vi "C-IV.vi"(5 "save?":bool=TRUE, 7 "Remote Lockin Address":string, 8 "error in":errorcluster, 9 "Experiment Comments":string="SA03036H\nsweep Vsg:-150mV to 600mV, 1mV steps\nB: 7T to -7T\nVbg = -3.9V\nT: 50mK\n\nlockin\n\nI+/-: 2/3 3mV ac+ 250uV dc bias, 0.4 Hz\nV1+/-: 8/4\nV2+/- 6/28\nV3+/V3-: 27/8\nVsg: 1\nVbg :26\n\ntc 300ms order 2", 10 "Experiment folder name":string="6H_IVcurves", 11 "SweepControl.lvclass":refnum<class "SweepControl.lvclass">) -> (0 "error out":errorcluster, 3 "SweepControl out":refnum<class "SweepControl.lvclass">)   [LabVIEW 2016, in "Transport.lvclass"]
uses:
  Transport.lvclass
  SweepControl/SweepControl.lvclass
  <userlib>/LevyLab/Lockin-Multichannel/Instrument.Lockin/Typedefs/AO-cluster.ctl
  <userlib>/LevyLab/Lockin-Multichannel/Instrument.Lockin/Typedefs/AO_Amp-array.ctl
  <userlib>/LevyLab/Lockin-Multichannel/Instrument.Lockin/Typedefs/AO_DC-array.ctl
  <userlib>/LevyLab/Lockin-Multichannel/Instrument.Lockin/Typedefs/AO_f-array.ctl
  <userlib>/LevyLab/Lockin-Multichannel/Instrument.Lockin/Typedefs/AO_phi-array.ctl
  <userlib>/LevyLab/Lockin-Multichannel/Instrument.Lockin/Typedefs/Function-array.ctl
  <userlib>/LevyLab/Lockin-Multichannel/Instrument.Lockin/Typedefs/Function-enum.ctl
  <userlib>/LevyLab/LV to ITX/LVtoITX.lvclass
  Control Experiment/Control Experiment.lvclass
  <userlib>/LevyLab/Lockin-Multichannel/Instrument.Lockin/Instrument.Lockin.lvclass
panel:
  out "4Term":cluster{dbl[], dbl[]}[](graph)
  out "2Term":T1(graph)
  in  "Tab Control":T2(tab)
  in  "Channels: AO":T3={"AO Amp (V)"=[0.01, 0.0, 0.0, 0.0, 0.0, 0.0, 0.0, 0.0], "AO DC (V)"=[0.0, 0.0, 0.0, 0.0, 0.0, 0.0, 0.0, 0.0], "AO f (Hz)"=[13.1, 13.0, 13.0, 13.0, 13.0, 13.0, 13.0, 13.0], "AO Phase (°)"=[0.0, 0.0, 0.0, 0.0, 0.0, 0.0, 0.0, 0.0], "Function"=[enum."Sine", enum."Sine", enum."Sine", enum."Sine", enum."Sine", enum."Sine", enum."Sine", enum."Sine"], "I+"=[], "Sweeping"=[]} {"AO f (Hz)" min=0.001 max=10000.0; "AO DC (V)" format="%.3p"; "AO Amp (V)" format="%.3p"}
  in  "Source Channel":i32
  in  "decimating factor":i32=1
  in  "low cutoff freq: fl":dbl=0.01 format="%0.4f"
  out "Temp":dbl
  in  "offset":dbl[](array[numeric])=[0.0, 0.0, 0.0, 0.0, 0.0, 0.0] format="%_6p"
  in  "invert":dbl[](array[numeric])=[1.0, 1.0, 1.0, 1.0, 1.0, 1.0] format="%#_6p"
  out "DC Voltages":dbl[](array[numeric])=[0.00025, 0.3, 0.0, 0.0, 0.0, 0.0, 0.0, 0.0, 0.00025, 0.3, 0.0, 0.0, 0.0, 0.0, 0.0, 0.0, 0.00025, 0.3, 0.0, 0.0, 0.0, 0.0, 0.0, 0.0, 0.00025, 0.3, 0.0, 0.0, 0.0, 0.0, 0.0, 0.0, 0.00025, 0.3, 0.0, 0.0, 0.0, 0.0, 0.0, 0.0, 0.00025, 0.3, 0.0, 0.0, 0.0, 0.0, 0.0, 0.0, 0.00025, 0.3, 0.0, 0.0, 0.0, 0.0, 0.0, 0.0, 0.00025, 0.3, 0.0, 0.0, 0.0, 0.0, 0.0, 0.0]
  out "Field (T)":dbl
  in  "Current":i32=1 min=1
  in  "V1":i32=1 min=1
  in  "V2":i32=1 min=1
  out "Input signal":waveform(dbl)[](graph)
  out "output":dbl[][](graph)
  # "CONFIGURE TO READ B FIELD AND TEMPERATURE!!!!"
  # "1"
  # "2"
  # "3"
  # "4"
  # "5"
  # "6"
  # "7"
  # "8"
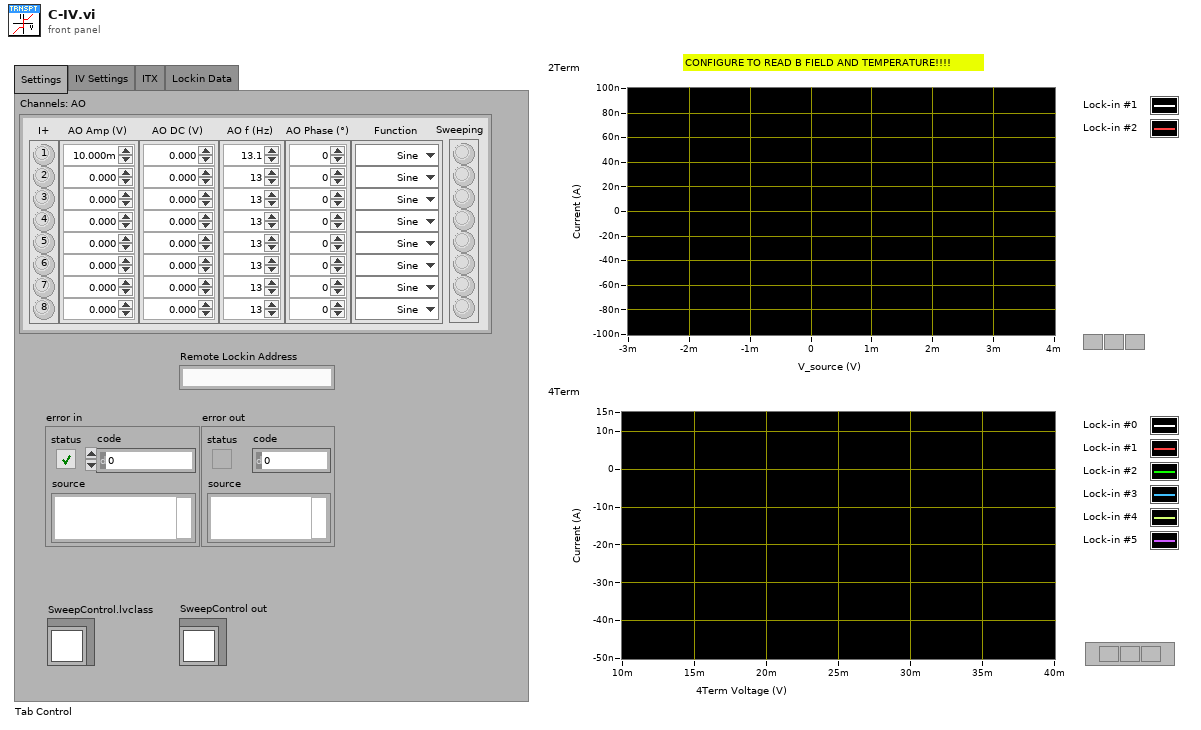
[diagram p1: front panel]
types:
  T1 = cluster{"Decimated and Filtered Array":dbl[], "Decimated and Filtered Array":dbl[]}[]
  T2 = enum32{"Settings", "IV Settings", "ITX", "Lockin Data"}
  T3 = typedef "Instrument.Lockin.lvclass/AO-cluster.ctl" = cluster{"AO Amp (V)":T4, "AO DC (V)":T5, "AO f (Hz)":T6, "AO Phase (°)":T7, "Function":T8, "I+":bool[], "Sweeping":bool[]}
  T4 = typedef "Instrument.Lockin.lvclass/AO_Amp-array.ctl" = dbl[]
  T5 = typedef "Instrument.Lockin.lvclass/AO_DC-array.ctl" = dbl[]
  T6 = typedef "Instrument.Lockin.lvclass/AO_f-array.ctl" = dbl[]
  T7 = typedef "Instrument.Lockin.lvclass/AO_phi-array.ctl" = dbl[]
  T8 = typedef "Instrument.Lockin.lvclass/Function-array.ctl" = T9[]
  T9 = typedef "Instrument.Lockin.lvclass/Function-enum.ctl" = enum16{"Sine", "Triangle", "Square", "Sawtooth"}
  T10 = cluster{"Decimated and Filtered Array":dbl[], "Decimated and Filtered Array":dbl[]}
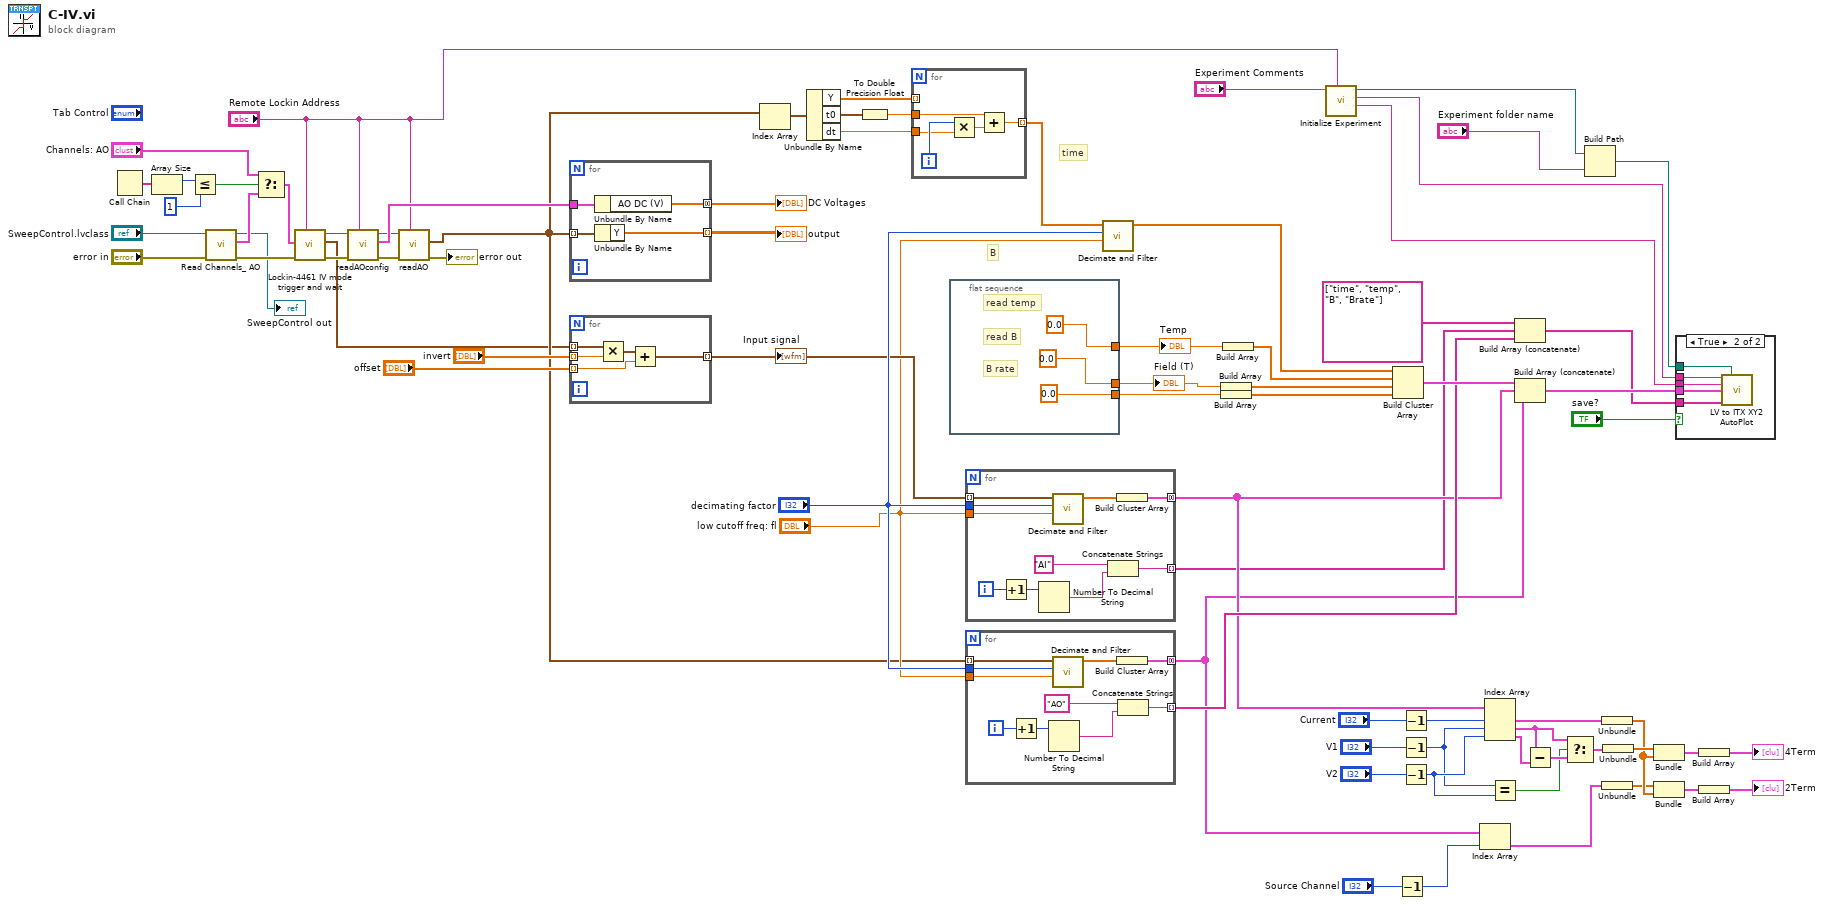
[diagram p0: block diagram]
diagram:
  # "time"
  # "B"
  n1 = Call Chain() -> (call chain=w35:string[])
  n2 = Array Size(array=w35) -> (size(s)=w34:i32)
  n3 = Less Or Equal?(x=w34, y=1) -> (x <= y?=w31:bool)
  n4 = call-dynamic "Read Channels_ AO.vi"("error in (no error)"="error in", "SweepControl in"="SweepControl.lvclass") -> ("error out"=w62:errorcluster, "Channels: AO"=w30:T3, "SweepControl out"=→"SweepControl out":refnum<class "SweepControl.lvclass">)  [unwired: 7 in]
  n5 = Select(t="Channels: AO", s=w31, f=w30) -> (s? t:f=w1:T3)
  n6 = call <userlib>:"Lockin-4461 IV mode trigger and wait.vi"("address"="Remote Lockin Address", "error in (no error)"=w62, "Channels: AO"=w1) -> ("error out"=w65:errorcluster, "input signal"=w4:waveform(dbl)[], "Instrument.Lockin out"=w3:refnum<class "Instrument.Lockin.lvclass">)  [unwired: 6 in]
  n7 = call <userlib>:"readAOconfig.vi"("address"="Remote Lockin Address", "error in (no error)"=w65, "Instrument.Lockin in"=w3) -> ("error out"=w66:errorcluster, "AOconfig"=w10:T3, "Instrument.Lockin out"=w2:refnum<class "Instrument.Lockin.lvclass">)  [unwired: 6 in]
  n8 = call <userlib>:"readAO.vi"("address"="Remote Lockin Address", "error in (no error)"=w66, "Instrument.Lockin in"=w2) -> ("error out"=→"error out":errorcluster, "output signal"=w9:waveform(dbl)[])  [unwired: 6 in, 1 out]
  n9 = for {
    tunnel: w9 -> [w81] mode=indexing
    tunnel: [w80] -> w77 mode=indexing
    tunnel: w10 -> [w79]
    tunnel: [w78] -> w53 mode=concatenating
    n10 = Unbundle By Name(w79) -> ("AO DC (V)"=w78:T5)
    n11 = Unbundle By Name(w81) -> ("Y"=w80:dbl[])
  }
  "output" <- w77
  "DC Voltages" <- w53
  n12 = for {
    tunnel: w4 -> [w85] mode=indexing
    tunnel: [w86] -> w12 mode=indexing
    tunnel: "offset" -> [w82] mode=indexing
    tunnel: "invert" -> [w84] mode=indexing
    n13 = Multiply(x=w85, y=w84) -> (x*y=w83:waveform(dbl))
    n14 = Add(x=w83, y=w82) -> (x+y=w86:waveform(dbl))
  }
  "Input signal" <- w12
  n15 = Index Array(array=w9) -> (element=w68:waveform(dbl))  [unwired: 1 in]
  n16 = Unbundle By Name(w68) -> ("Y"=w67:dbl[], "t0"=w69:timestamp, "dt"=w70:dbl)
  n17 = To Double Precision Float(number=w69) -> (double precision float=w71:dbl)
  n18 = for {
    tunnel: w70 -> [w90]
    tunnel: w71 -> [w88]
    tunnel: [w87] -> w27 mode=indexing
    tunnel: w67 -> [_] mode=indexing
    i -> [w91]
    n19 = Multiply(x=w91, y=w90) -> (x*y=w89:dbl)
    n20 = Add(x=w88, y=w89) -> (x+y=w87:dbl)
  }
  n21 = flat-sequence {
    tunnel: [0.0 ("element")] -> w54
    tunnel: [0.0] -> w8
    tunnel: [0.0 ("element")] -> w7
    frame #0 {
      # "read B"
      # "read temp"
      # "B rate"
    }
  }
  n22 = for {
    tunnel: "low cutoff freq: fl" -> [w95]
    tunnel: w12 -> [w104] mode=indexing
    tunnel: [w98] -> w16 mode=concatenating
    tunnel: [w97] -> w15 mode=indexing
    tunnel: "decimating factor" -> [w96]
    i -> [w100]
    n23 = Increment(x=w100) -> (x+1=w103:i32)
    n24 = Number To Decimal String(number=w103) -> (decimal integer string=w102:string)  [unwired: 1 in]
    n25 = call "Decimate and Filter.vi"("low cutoff freq: fl"=w95, "decimating factor"=w96, "Waveform in"=w104) -> ("Decimated and Filtered Array"=w99:dbl[])  [unwired: 7 in, 1 out]
    n26 = Concatenate Strings("AI" ("wavenames"), w102) -> (w97:string)
    n27 = Build Cluster Array(w99) -> (w98:cluster{"Decimated and Filtered Array":dbl[]}[])
  }
  n28 = for {
    tunnel: "low cutoff freq: fl" -> [w105]
    tunnel: w9 -> [w114] mode=indexing
    tunnel: [w108] -> w14 mode=concatenating
    tunnel: [w107] -> w29 mode=indexing
    tunnel: "decimating factor" -> [w106]
    i -> [w110]
    n29 = Increment(x=w110) -> (x+1=w113:i32)
    n30 = Number To Decimal String(number=w113) -> (decimal integer string=w112:string)  [unwired: 1 in]
    n31 = call "Decimate and Filter.vi"("low cutoff freq: fl"=w105, "decimating factor"=w106, "Waveform in"=w114) -> ("Decimated and Filtered Array"=w109:dbl[])  [unwired: 7 in, 1 out]
    n32 = Build Cluster Array(w109) -> (w108:cluster{"Decimated and Filtered Array":dbl[]}[])
    n33 = Concatenate Strings("AO" ("wavenames"), w112) -> (w107:string)
  }
  n34 = call "Decimate and Filter.vi"("low cutoff freq: fl"="low cutoff freq: fl", "decimating factor"="decimating factor", "Waveform in"=w27) -> ("Decimated and Filtered Array"=w26:dbl[])  [unwired: 7 in, 1 out]
  n35 = Build Array(w7) -> (w58:dbl[])
  n36 = Build Array(w54) -> (w55:dbl[])
  n37 = Build Array(w8) -> (w59:dbl[])
  n38 = call "Initialize Experiment.vi"("lockin address"="Remote Lockin Address", "Experiment Comments"="Experiment Comments") -> ("Comments"=w13:string, "device"=w37:string, "path"=w39:path)  [unwired: 6 in, 1 out]
  n39 = Build Cluster Array(w26, w59, w58, w55) -> (w57:cluster{"Decimated and Filtered Array":dbl[]}[])
  n40 = Decrement(x="Source Channel") -> (x-1=w20:i32)
  n41 = Decrement(x="Current") -> (x-1=w48:i32)
  n42 = Decrement(x="V1") -> (x-1=w24:i32)
  n43 = Decrement(x="V2") -> (x-1=w45:i32)
  n44 = Index Array(array=w14, index=w20) -> (element=w19:cluster{"Decimated and Filtered Array":dbl[]})
  n45 = Index Array(array=w16, index #1=w48, index #2=w24, index #3=w45) -> (element #1=w42:cluster{"Decimated and Filtered Array":dbl[]}, element #2=w46:cluster{"Decimated and Filtered Array":dbl[]}, element #3=w40:cluster{"Decimated and Filtered Array":dbl[]})
  n46 = Equal?(x=w24, y=w45) -> (x = y?=w44:bool)
  n47 = Build Array (concatenate)(string[] ["time", "temp", "B", "Brate"] ("wavenames (.Vx, etc)"), w15, w29) -> (w51:string[])
  n48 = Build Array (concatenate)(w57, w16, w14) -> (w52:cluster{"Decimated and Filtered Array":dbl[]}[])
  n49 = Subtract(x=w46, y=w40) -> (x-y=w47:cluster{"Decimated and Filtered Array":dbl[]})
  n50 = Select(t=w46, s=w44, f=w47) -> (s? t:f=w43:cluster{"Decimated and Filtered Array":dbl[]})
  n51 = Build Path(base path=w39, name or relative path="Experiment folder name") -> (appended path=w76:path)
  n52 = Unbundle(w42) -> ("Decimated and Filtered Array"=w22:dbl[])
  n53 = Unbundle(w19) -> ("Decimated and Filtered Array"=w21:dbl[])
  n54 = Unbundle(w43) -> ("Decimated and Filtered Array"=w41:dbl[])
  n55 = Bundle("Decimated and Filtered Array"=w41, "Decimated and Filtered Array"=w22) -> (w75:T10)  [unwired: 1 in]
  n56 = Bundle("Decimated and Filtered Array"=w21, "Decimated and Filtered Array"=w22) -> (w18:T10)  [unwired: 1 in]
  n57 = case shown="True" "save?" {
    tunnel: w76 -> [_ w119]
    tunnel: w37 -> [_ w118]
    tunnel: w13 -> [_ w117]
    tunnel: w52 -> [_ w116]
    tunnel: w51 -> [_ w115]
    frame False {
    }
    frame True {
      n58 = call <userlib>:"LV to ITX XY2 AutoPlot.vi"("filename"=w118, "path"=w119, "Notes"=w117, "Data"=w116, "wavenames (.Vx, etc)"=w115) -> ()  [unwired: 10 in, 1 out]
    }
  }
  n59 = Build Array(w75) -> (→"4Term":T1)
  n60 = Build Array(w18) -> (→"2Term":T1)
  "Temp" <- w8
  "Field (T)" <- w7
